vi "Read Message Type and Terminals.vi"(8 "error in":errorcluster, 11 "message ref in":refnum<k20>) -> (0 "error out":errorcluster, 1 "mode code":u16, 2 "message type":T3, 3 "message ref out":refnum<k20>, 4 "Rx terminal":T1, 6 "Tx terminal":T1)   [LabVIEW 2020, in "MIL-STD 1553 Import.lvlib"]
uses:
  MIL-STD 1553 Import.lvlib
  Shared/Message Type.ctl
  Shared/Terminal Endpoint.ctl
  Shared/Address.ctl
  be799091-bce2-4db8-b401-a39db5fe7e6e.vi
  7b932162-56eb-46b3-8687-de5d8e1261b8.vi
  660cc6a3-cbfa-43c5-9af2-575de6bf616f.vi
  40e07135-e19e-4b22-895a-2c183958625d.vi/f2e36f1e-2f32-4ca0-af02-7f64f8835cd4.vi
  3546f335-97ce-4ffc-962d-2f5ff9bf87c1.vi/a680c3a9-01fa-4afe-b51c-d70142d2274f.vi
  487ea7c7-ffca-4428-88f2-a900c8ae7e8d.vi/83528eed-c3c3-41f2-8a2d-c4938446405f.vi
  3546f335-97ce-4ffc-962d-2f5ff9bf87c1.vi/b1e6fcf8-dac1-42d2-b1fe-151afe06dbd4.vi/132e18cf-dd6f-4d74-b273-c733e0aa38c6.vi
  Constants.vi
  <vilib>/xml/Get Node Text Content.vi
  <vilib>/Utility/error.llb/Error Cluster From Error Code.vi
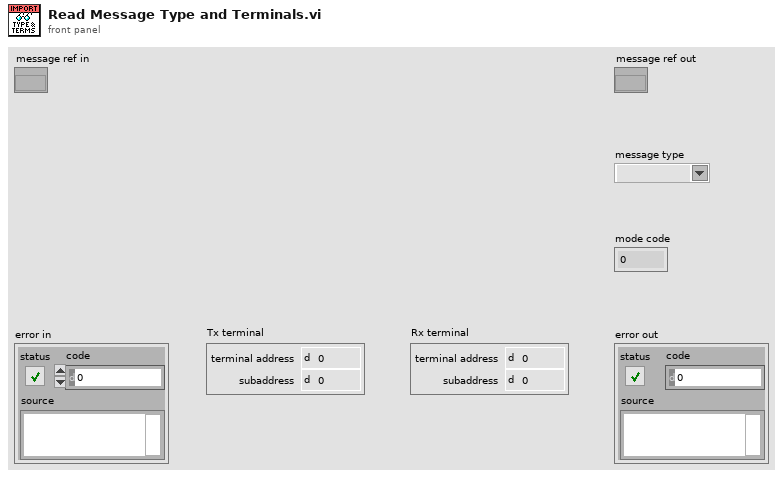
[diagram p1: front panel]
types:
  T1 = typedef "Terminal Endpoint.ctl" = cluster{"terminal address":T2, "subaddress":T2}
  T2 = typedef "Address.ctl" = u16
  T3 = typedef "Message Type.ctl" = string
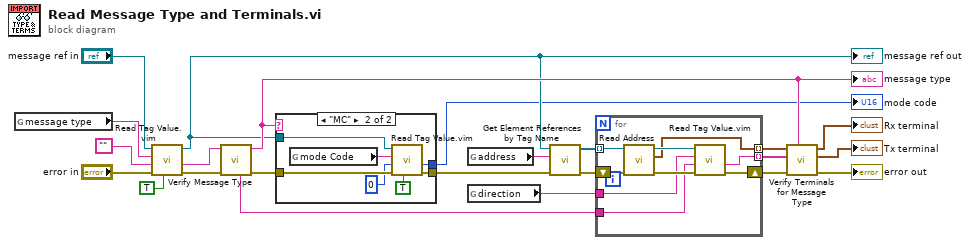
[diagram p0: block diagram]
diagram:
  n1 = global read "Constants.vi" "message type"() -> (w23:string)
  n2 = call "Read Tag Value.vim"("required (F)"=TRUE, "error in"="error in", "default"="", "tag name"=w23, "node in"="message ref in") -> ("error out"=w19:errorcluster, "value"=w18:string, "node out"=w2:refnum<k20>)  [unwired: 4 in]
  "message ref out" <- w2
  n3 = call "Verify Message Type.vi"("error in"=w19, "message type in"=w18) -> ("error out"=w5:errorcluster, "message type out"=w3:T3, "expected RT direction"=w6:string)  [unwired: 6 in, 1 out]
  "message type" <- w3
  n4 = case shown="\"MC\"" w3 {
    tunnel: w5 -> [w24 w31]
    tunnel: [w24 w30] -> w4
    tunnel: w2 -> [_ w26]
    tunnel: [_ w25] -> w1
    frame Default {
    }
    frame "MC" {
      n5 = global read "Constants.vi" "mode Code"() -> (w27:string)
      n6 = call "Read Tag Value.vim"("required (F)"=TRUE, "error in"=w31, "default"=u16 0, "tag name"=w27, "node in"=w26) -> ("error out"=w30:errorcluster, "value"=w25:u16)  [unwired: 4 in, 1 out]
    }
  }
  "mode code" <- w1
  n7 = global read "Constants.vi" "address"() -> (w17:string)
  n8 = global read "Constants.vi" "direction"() -> (w14:string)
  n9 = call "Get Element References by Tag Name.vi"("error in"=w4, "tag name"=w17, "node in"=w2) -> ("error out"=w16:errorcluster, "array of elements"=w15:refnum<k20>[])  [unwired: 7 in]
  n10 = for {
    shift-right: [w38] -> w13
    shift-left: w16 -> [w40]
    tunnel: w15 -> [w37] mode=indexing
    tunnel: w14 -> [w35]
    tunnel: w6 -> [w34]
    tunnel: [w33] -> w10 mode=indexing
    tunnel: [w32] -> w9 mode=indexing
    n11 = call "Read Address.vi"("error in"=w40, "address ref in"=w37) -> ("error out"=w39:errorcluster, "terminal"=w32:T1, "address ref out"=w36:refnum<k20>)  [unwired: 7 in]
    n12 = call "Read Tag Value.vim"("error in"=w39, "default"=w34, "tag name"=w35, "node in"=w36) -> ("error out"=w38:errorcluster, "value"=w33:string)  [unwired: 5 in, 1 out]
  }
  n13 = call "Verify Terminals for Message Type.vi"("message type"=w3, "error in"=w13, "directions"=w10, "terminals"=w9) -> ("error out"=→"error out":errorcluster, "Tx terminal"=→"Tx terminal":T1, "Rx terminal"=→"Rx terminal":T1)  [unwired: 5 in]
